vi "Temperature Monitor.vi"() -> ()   [LabVIEW 2018]
doc: "This VI is the solution to an exercise in the LabVIEW Core 1 course.\n\nIt uses a While Loop and shift registers to average data. No hardware is necessary."
panel:
  out "x/y":dbl
  in  "Stop Button":bool
  out "Temperature History":dbl(graph)
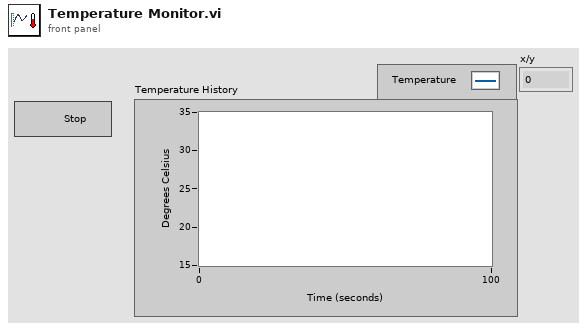
[diagram p1: front panel]
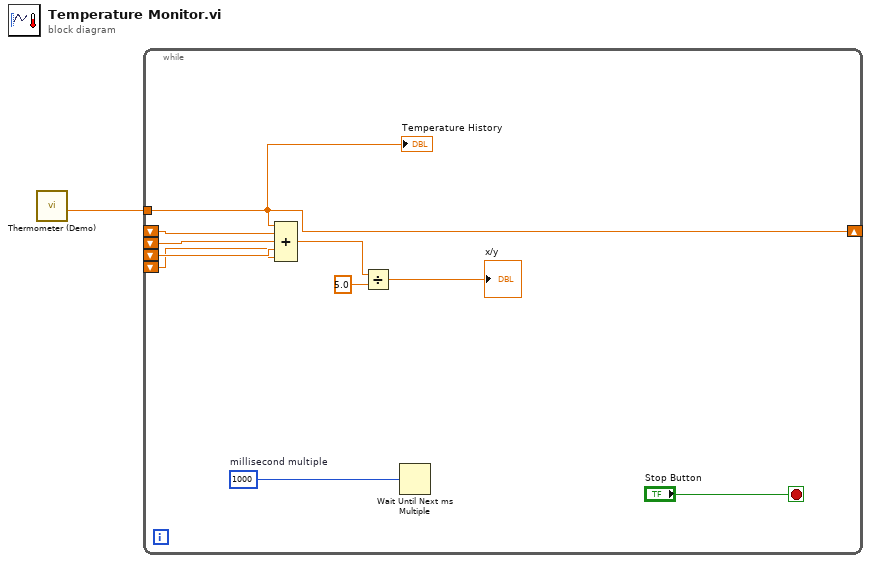
[diagram p0: block diagram]
diagram:
  n1 = call "Thermometer (Demo).vi"() -> ("Temperature Value"=w1:dbl)  [unwired: 11 in]
  n2 = while {
    shift-right: [w2] -> _
    shift-left: _ -> [w9]
    shift-left: _ -> [w8]
    shift-left: _ -> [w7]
    shift-left: _ -> [w6]
    tunnel: w1 -> [w2]
    stop <- "Stop Button" stop-if-true
    w11 = u32 1000  # millisecond multiple
    n3 = Compound Arithmetic op=ADD(w2, w9, w8, w7, w6) -> (w4:dbl)
    n4 = Divide(x=w4, y=5.0) -> (x/y=→"x/y":dbl)
    n5 = Wait Until Next ms Multiple(millisecond multiple=w11) -> ()  [unwired: 1 out]
    "Temperature History" <- w2
  }
